vi "ELVIS III v1.0 Build MUX Configuration AO Block.vi"(11 "AO (N Samples) Channels List":T4) -> (2 "AIO Mode bitmask":bool[][](array[boolean]), 3 "Channel Reservation Info":T1)   [LabVIEW 2021]
uses:
  <vilib>/myRIO/Common/Instrument Driver Framework/myRIO v1.0/AO Block/typedefs/AO Block Channels List.ctl
  <vilib>/myRIO/Common/Instrument Driver Framework/myRIO v1.0/AO Block/typedefs/AO Block Channels Enum.ctl
  <vilib>/myRIO/Common/Instrument Driver Framework/ELVIS III v1.0/Resource Manager/typedefs/ELVIS III v1.0 Channel Reservation List.ctl
  <vilib>/myRIO/Common/Instrument Driver Framework/ELVIS III v1.0/Resource Manager/typedefs/ELVIS III v1.0 Channel Reservation Info.ctl
  <vilib>/myRIO/Common/Instrument Driver Framework/ELVIS III v1.0/Resource Manager/typedefs/ELVIS III v1.0 Connector List.ctl
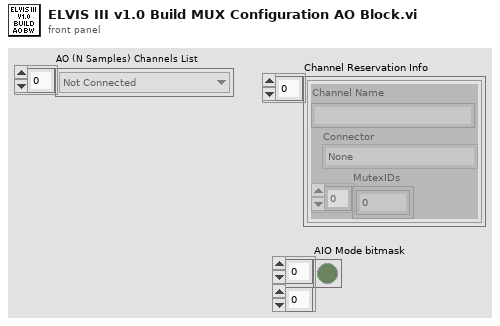
[diagram p1: front panel]
types:
  T1 = typedef "ELVIS III v1.0 Channel Reservation List.ctl" = T2[]
  T2 = typedef "ELVIS III v1.0 Channel Reservation Info.ctl" = cluster{"Channel Name":string, "Connector":T3, "MutexIDs":u32[]}
  T3 = typedef "ELVIS III v1.0 Connector List.ctl" = enum32{"None", "ConnectorA", "ConnectorB"}
  T4 = typedef "AO Block Channels List.ctl" = T5[]
  T5 = typedef "AO Block Channels Enum.ctl" = enum16{"Not Connected", "A/AO0 (N Samples)", "A/AO1 (N Samples)", "B/AO0 (N Samples)", "B/AO1 (N Samples)"}
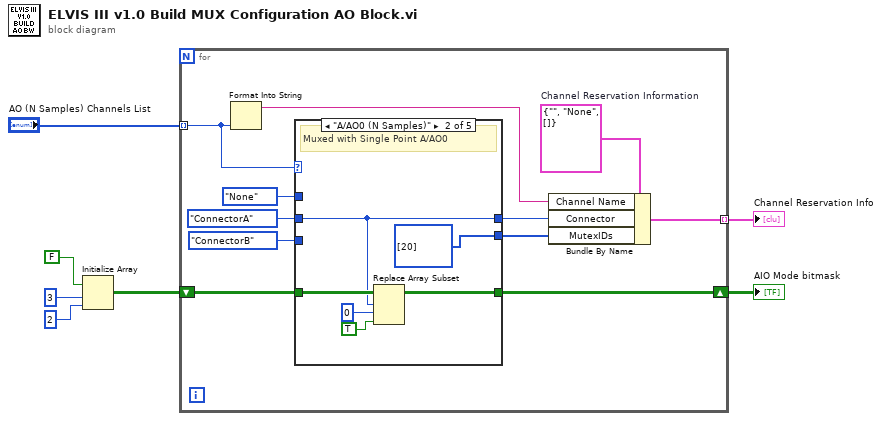
[diagram p0: block diagram]
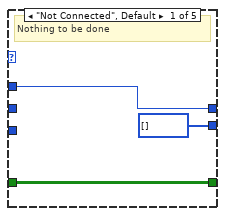
[diagram p2: hidden frame]
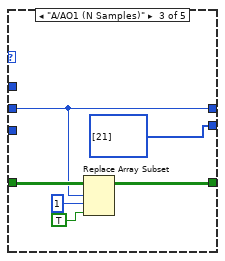
[diagram p3: hidden frame]
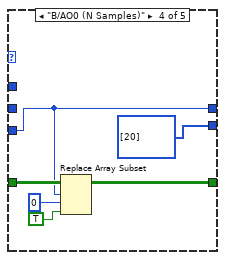
[diagram p4: hidden frame]
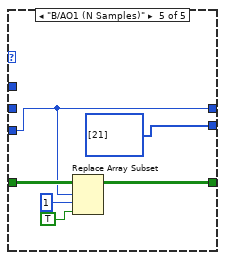
[diagram p5: hidden frame]
diagram:
  n1 = Initialize Array(FALSE, 3 ("dimension size"), 2 ("dimension size")) -> (w2:bool[][])
  n2 = for {
    tunnel: "AO (N Samples) Channels List" -> [w15] mode=indexing
    tunnel: [w16] -> w6 mode=indexing
    shift-right: [w8] -> w1
    shift-left: w2 -> [w9]
    w18 = T2 {"Channel Name"="", "Connector"=enum."None", "MutexIDs"=[]}  # Channel Reservation Information
    n3 = Format Into String(w15) -> (resulting string=w17:string)  [unwired: 3 in, 1 out]
    n4 = case shown="\"A/AO0 (N Samples)\"" w15 {
      tunnel: ELVIS_III_v1.0_Connector_List."None" ("Connector") -> [w21 _ _ _ _]
      tunnel: [w21 w23 w28 w34 w40] -> w13
      tunnel: ELVIS_III_v1.0_Connector_List."ConnectorA" ("Connector") -> [_ w23 w28 _ _]
      tunnel: ELVIS_III_v1.0_Connector_List."ConnectorB" ("Connector") -> [_ _ _ w34 w40]
      tunnel: [u32[] [] ("MutexIDs") u32[] [20] ("MutexIDs") u32[] [21] ("MutexIDs") u32[] [20] ("MutexIDs") u32[] [21] ("MutexIDs")] -> w10
      tunnel: w9 -> [w19 w24 w30 w36 w42]
      tunnel: [w19 w22 w29 w35 w41] -> w8
      frame "Not Connected", Default {
        # "Nothing to be done"
      }
      frame "A/AO0 (N Samples)" {
        # "Muxed with Single Point A/AO0"
        n5 = Replace Array Subset(array=w24, new element=TRUE ("new element/subarray"), index (row)=w23, index (col)=0 ("disabled index (col)")) -> (w22:bool[][])
      }
      frame "A/AO1 (N Samples)" {
        n6 = Replace Array Subset(array=w30, new element=TRUE ("new element/subarray"), index (row)=w28, index (col)=1 ("disabled index (col)")) -> (w29:bool[][])
      }
      frame "B/AO0 (N Samples)" {
        n7 = Replace Array Subset(array=w36, new element=TRUE ("new element/subarray"), index (row)=w34, index (col)=0 ("disabled index (col)")) -> (w35:bool[][])
      }
      frame "B/AO1 (N Samples)" {
        n8 = Replace Array Subset(array=w42, new element=TRUE ("new element/subarray"), index (row)=w40, index (col)=1 ("disabled index (col)")) -> (w41:bool[][])
      }
    }
    n9 = Bundle By Name(cluster=w18, "Channel Name"=w17, "Connector"=w13, "MutexIDs"=w10) -> (w16:T2)
  }
  "Channel Reservation Info" <- w6
  "AIO Mode bitmask" <- w1
